vi "Fancy Dance.vi"   [LabVIEW 2013]
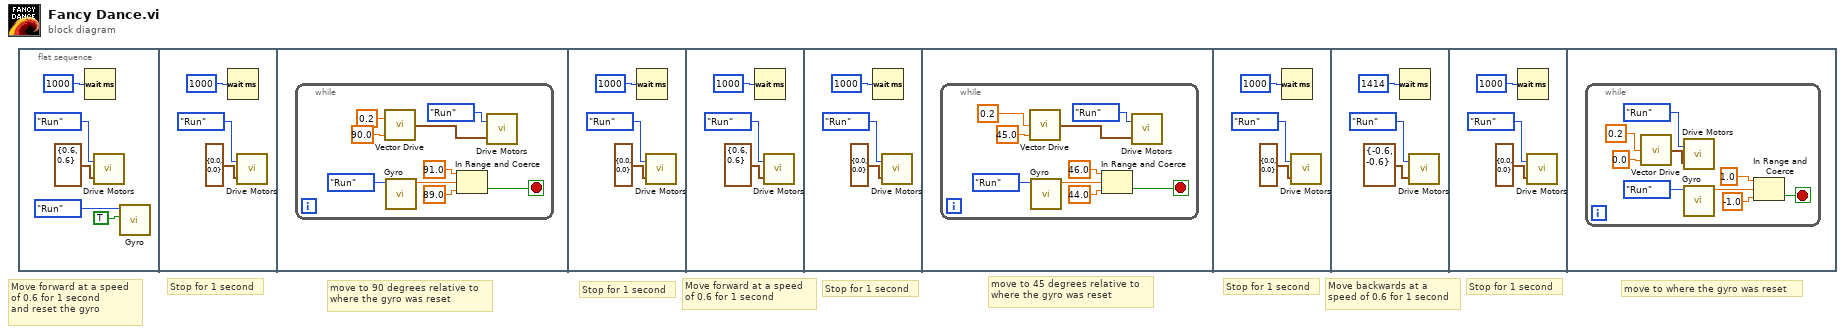
[diagram p0: block diagram]
diagram:
  # "move to where the gyro was reset"
  # "Move backwards at a \nspeed of 0.6 for 1 second"
  # "Stop for 1 second"
  # "Stop for 1 second"
  # "move to 45 degrees relative to \nwhere the gyro was reset"
  # "Stop for 1 second"
  # "Move forward at a speed\nof 0.6 for 1 second"
  # "Stop for 1 second"
  # "move to 90 degrees relative to \nwhere the gyro was reset"
  # "Stop for 1 second"
  # "Move forward at a speed\nof 0.6 for 1 second\nand reset the gyro"
  n1 = flat-sequence {
    frame #0 {
      n2 = Wait (ms)(milliseconds to wait=u32 1000) -> ()  [unwired: 1 out]
      n3 = call "Drive Motors.vi"("Motor Powers"=cluster{"RMotor":dbl, "LMotor":dbl} {"RMotor"=0.6, "LMotor"=0.6}, "Enum"=enum16{"Start", "Run", "End"}."Run") -> ()
      n4 = call "Gyro.vi"("Reset"=TRUE, "Enum"=enum16{"Start", "Run", "End"}."Run") -> ()  [unwired: 9 in, 1 out]
    }
    frame #1 {
      n5 = Wait (ms)(milliseconds to wait=u32 1000) -> ()  [unwired: 1 out]
      n6 = call "Drive Motors.vi"("Motor Powers"=cluster{"RMotor":dbl, "LMotor":dbl} {"RMotor"=0.0, "LMotor"=0.0}, "Enum"=enum16{"Start", "Run", "End"}."Run") -> ()
    }
    frame #2 {
      n7 = while {
        stop <- w10 stop-if-true
        n8 = call "Vector Drive.vi"("Angle"=90.0, "Min. Power"=0.2) -> ("Motor Powers"=w16:cluster{"RMotor":dbl, "LMotor":dbl})  [unwired: 1 in]
        n9 = call "Gyro.vi"("Enum"=enum16{"Start", "Run", "End"}."Run") -> ("Angle"=w13:dbl)  [unwired: 10 in]
        n10 = In Range and Coerce(upper limit=91.0 ("Angle"), x=w13, lower limit=89.0 ("Angle")) -> (In Range?=w10:bool)  [unwired: 1 out]
        n11 = call "Drive Motors.vi"("Motor Powers"=w16, "Enum"=enum16{"Start", "Run", "End"}."Run") -> ()
      }
    }
    frame #3 {
      n12 = Wait (ms)(milliseconds to wait=u32 1000) -> ()  [unwired: 1 out]
      n13 = call "Drive Motors.vi"("Motor Powers"=cluster{"RMotor":dbl, "LMotor":dbl} {"RMotor"=0.0, "LMotor"=0.0}, "Enum"=enum16{"Start", "Run", "End"}."Run") -> ()
    }
    frame #4 {
      n14 = Wait (ms)(milliseconds to wait=u32 1000) -> ()  [unwired: 1 out]
      n15 = call "Drive Motors.vi"("Motor Powers"=cluster{"RMotor":dbl, "LMotor":dbl} {"RMotor"=0.6, "LMotor"=0.6}, "Enum"=enum16{"Start", "Run", "End"}."Run") -> ()
    }
    frame #5 {
      n16 = Wait (ms)(milliseconds to wait=u32 1000) -> ()  [unwired: 1 out]
      n17 = call "Drive Motors.vi"("Motor Powers"=cluster{"RMotor":dbl, "LMotor":dbl} {"RMotor"=0.0, "LMotor"=0.0}, "Enum"=enum16{"Start", "Run", "End"}."Run") -> ()
    }
    frame #6 {
      n18 = while {
        stop <- w28 stop-if-true
        n19 = call "Vector Drive.vi"("Angle"=45.0, "Min. Power"=0.2) -> ("Motor Powers"=w34:cluster{"RMotor":dbl, "LMotor":dbl})  [unwired: 1 in]
        n20 = call "Gyro.vi"("Enum"=enum16{"Start", "Run", "End"}."Run") -> ("Angle"=w31:dbl)  [unwired: 10 in]
        n21 = In Range and Coerce(upper limit=46.0 ("Angle"), x=w31, lower limit=44.0 ("Angle")) -> (In Range?=w28:bool)  [unwired: 1 out]
        n22 = call "Drive Motors.vi"("Motor Powers"=w34, "Enum"=enum16{"Start", "Run", "End"}."Run") -> ()
      }
    }
    frame #7 {
      n23 = Wait (ms)(milliseconds to wait=u32 1000) -> ()  [unwired: 1 out]
      n24 = call "Drive Motors.vi"("Motor Powers"=cluster{"RMotor":dbl, "LMotor":dbl} {"RMotor"=0.0, "LMotor"=0.0}, "Enum"=enum16{"Start", "Run", "End"}."Run") -> ()
    }
    frame #8 {
      n25 = Wait (ms)(milliseconds to wait=u32 1414) -> ()  [unwired: 1 out]
      n26 = call "Drive Motors.vi"("Motor Powers"=cluster{"RMotor":dbl, "LMotor":dbl} {"RMotor"=-0.6, "LMotor"=-0.6}, "Enum"=enum16{"Start", "Run", "End"}."Run") -> ()
    }
    frame #9 {
      n27 = Wait (ms)(milliseconds to wait=u32 1000) -> ()  [unwired: 1 out]
      n28 = call "Drive Motors.vi"("Motor Powers"=cluster{"RMotor":dbl, "LMotor":dbl} {"RMotor"=0.0, "LMotor"=0.0}, "Enum"=enum16{"Start", "Run", "End"}."Run") -> ()
    }
    frame #10 {
      n29 = while {
        stop <- w46 stop-if-true
        n30 = call "Vector Drive.vi"("Angle"=0.0, "Min. Power"=0.2) -> ("Motor Powers"=w52:cluster{"RMotor":dbl, "LMotor":dbl})  [unwired: 1 in]
        n31 = call "Drive Motors.vi"("Motor Powers"=w52, "Enum"=enum16{"Start", "Run", "End"}."Run") -> ()
        n32 = call "Gyro.vi"("Enum"=enum16{"Start", "Run", "End"}."Run") -> ("Angle"=w49:dbl)  [unwired: 10 in]
        n33 = In Range and Coerce(upper limit=1.0 ("Angle"), x=w49, lower limit=-1.0 ("Angle")) -> (In Range?=w46:bool)  [unwired: 1 out]
      }
    }
  }
